vi "Check Tree Item Icon.vi"(0 "TreeControl in":refnum<vi>, 5 "Active Item Tag":string, 11 "error in (no error)":errorcluster) -> (4 "TreeControl out":refnum<vi>, 6 "Valid symbol?":bool, 15 "error out":errorcluster)   [LabVIEW 2021, in "Converter.lvlib"]
uses:
  Converter.lvlib
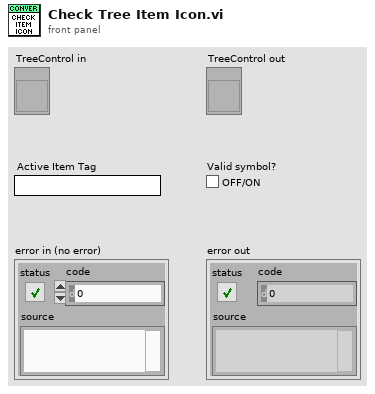
[diagram p1: front panel]
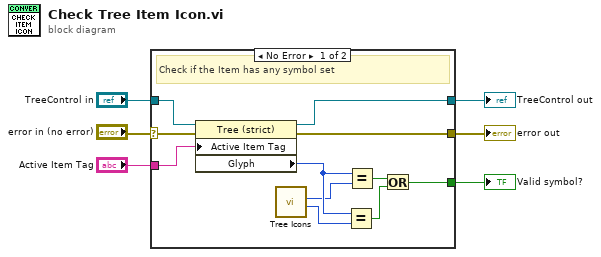
[diagram p0: block diagram]
diagram:
  n1 = case shown="No Error" "error in (no error)" {
    selector: "error in (no error)" -> [w8 w18]
    tunnel: [w17 w19] -> w6
    tunnel: [w16 w18] -> w5
    tunnel: [w14 _] -> w4
    tunnel: "TreeControl in" -> [w13 w19]
    tunnel: "Active Item Tag" -> [w7 _]
    frame No Error {
      # "Check if the Item has any symbol set"
      n2 = property on="Property Node" class="Tree (strict)"(reference=w13, error in=w8, "Active Item Tag"=w7) -> (reference out=w17:refnum<vi>, error out=w16:errorcluster, "Glyph"=w15:i32)
      n3 = call "Tree Icons.vi"() -> ("Not Selected"=w10:i32, "Selected"=w9:i32)  [unwired: 6 in]
      n4 = Equal?(x=w15, y=w10) -> (x = y?=w12:bool)
      n5 = Equal?(x=w15, y=w9) -> (x = y?=w11:bool)
      n6 = Or(x=w11, y=w12) -> (x .or. y?=w14:bool)
    }
    frame Error {
      # "Pass"
    }
  }
  "TreeControl out" <- w6
  "error out" <- w5
  "Valid symbol?" <- w4
